vi "PMLambda-Conct Rev B.vi"(0 "FW inTest":u16(ring) items=["WSD Board", "NML Board"], 2 "work buffer":string, 5 "error in":errorcluster, 6 "Supply Cnt":i32=1 min=1 max=5 step=1, 7 "N Systems":i32=1 min=1 max=8 step=1, 8 "COM Ref In":refnum<vi>, 10 "Msg Ref In":refnum<vi>, 11 "Loop Index":i32) -> (14 "Re-conf Lambda?":bool, 15 "Lambda, nm":i32, 19 "error out":errorcluster)   [LabVIEW 2017]
panel:
  # "Inputs"
  # "Outputs"
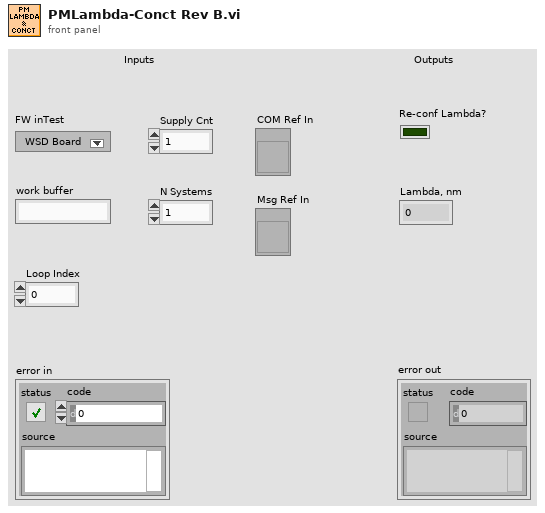
[diagram p1: front panel]
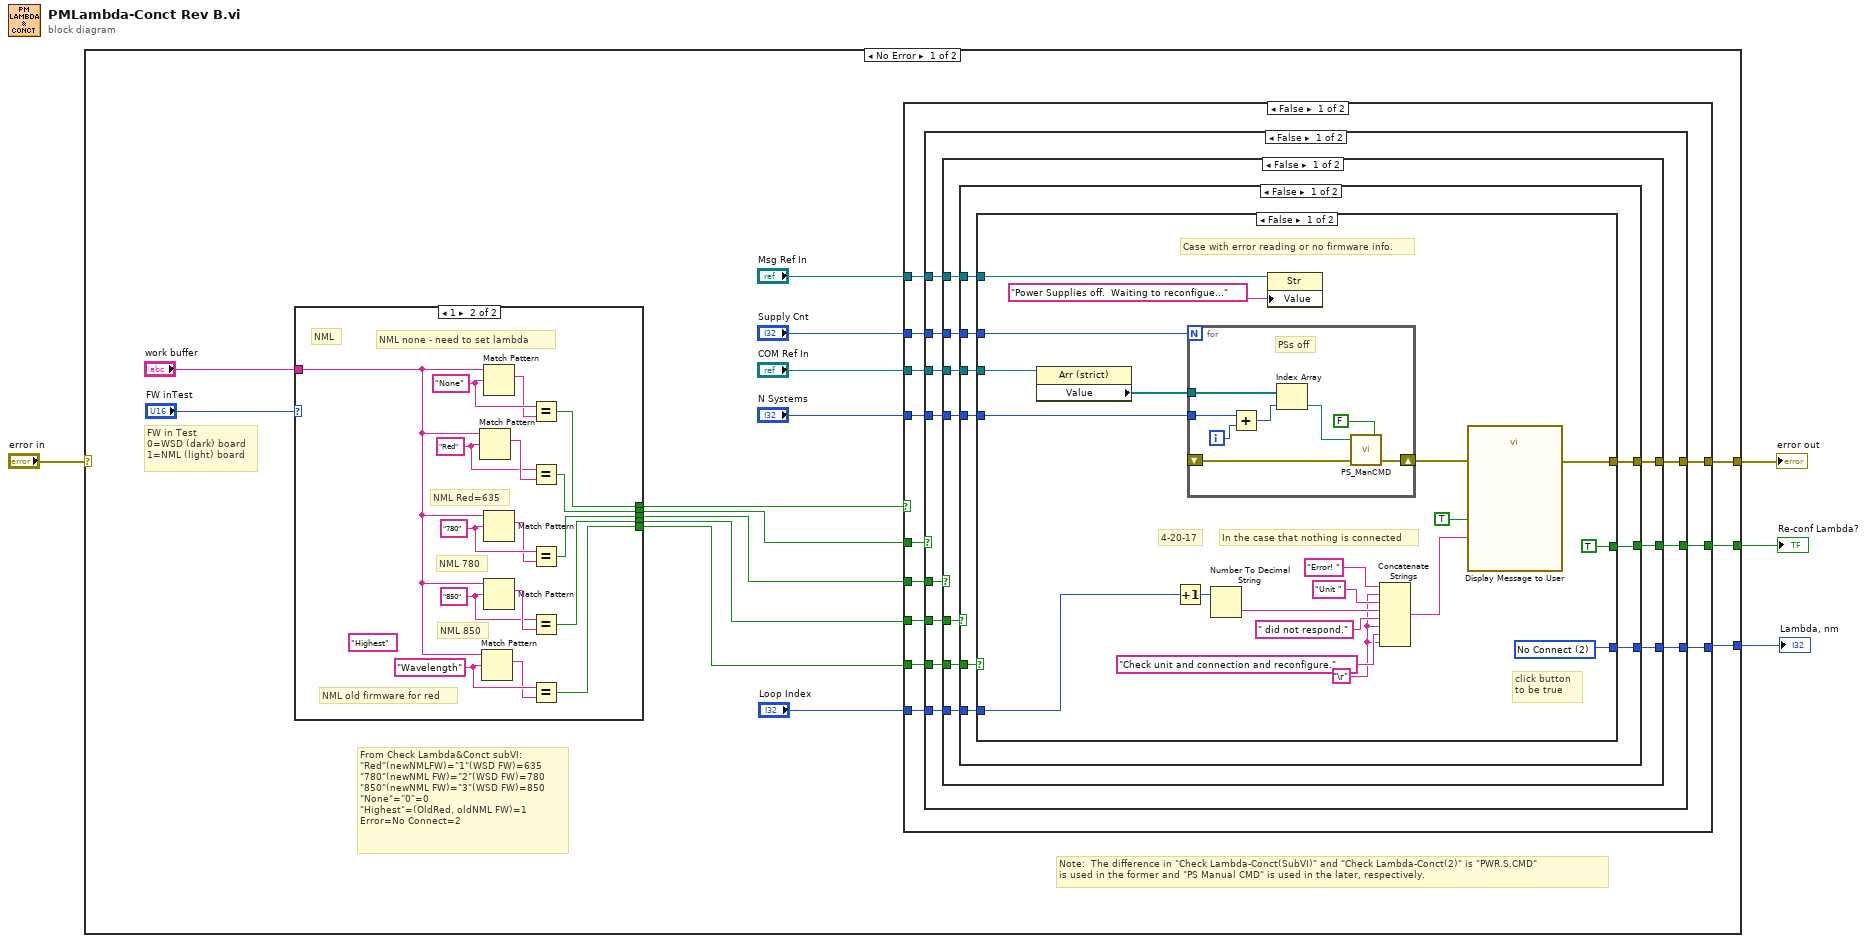
[diagram p0: block diagram]
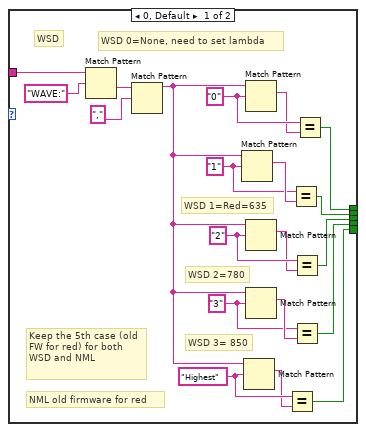
[diagram p2: hidden frame]
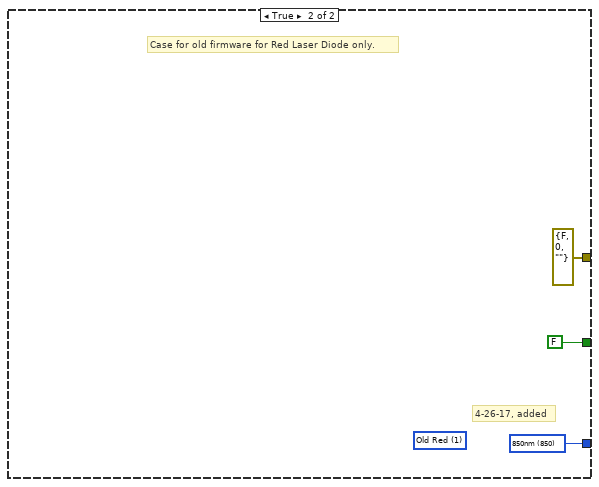
[diagram p3: hidden frame]
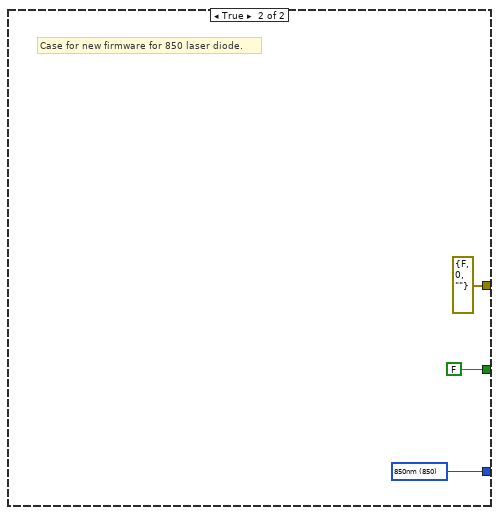
[diagram p4: hidden frame]
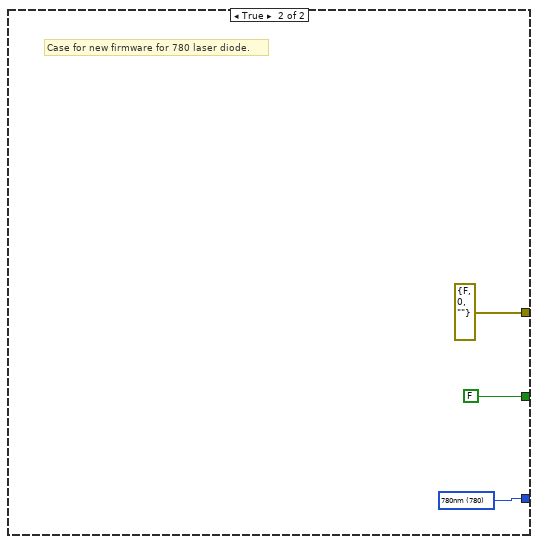
[diagram p5: hidden frame]
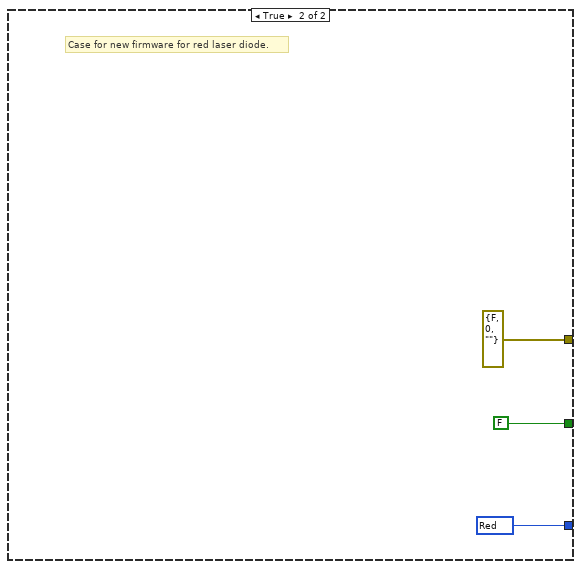
[diagram p6: hidden frame]
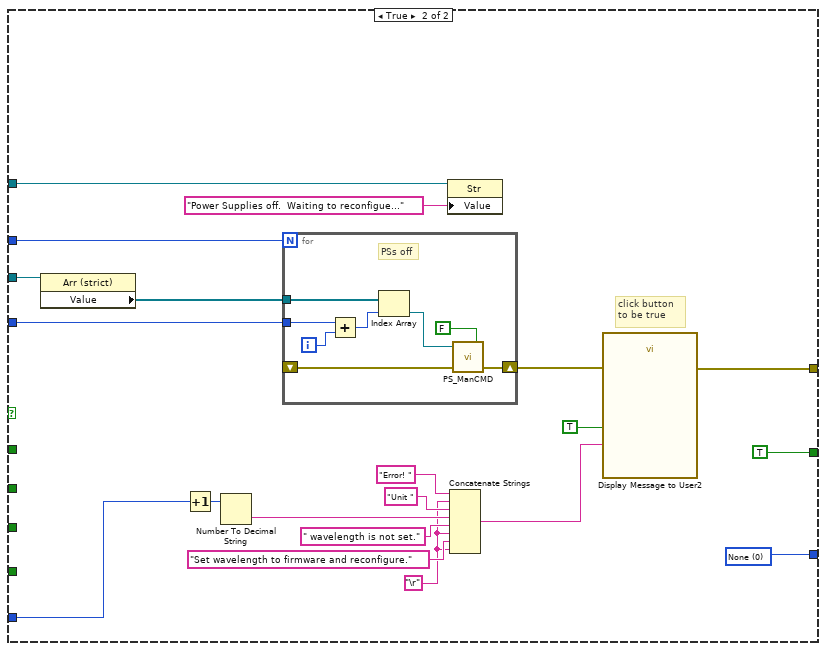
[diagram p7: hidden frame]
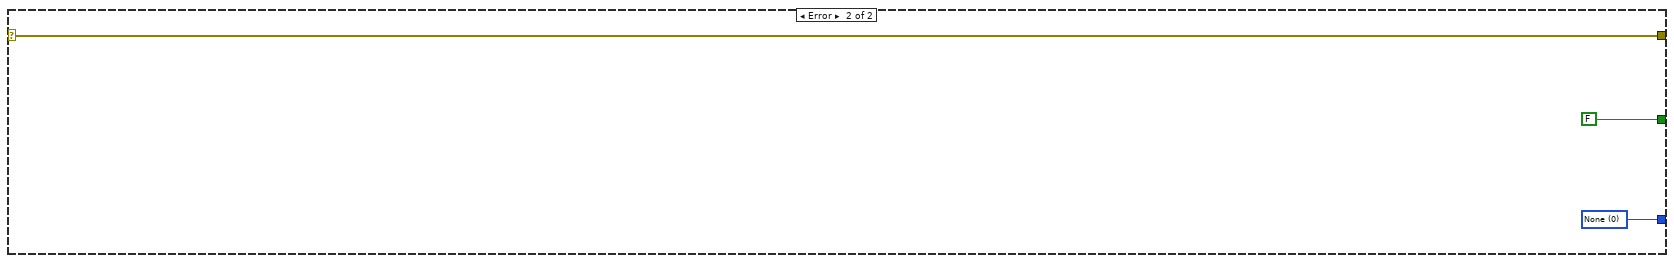
[diagram p8: hidden frame]
diagram:
  n1 = case shown="No Error" "error in" {
    selector: "error in" -> [_ w168]
    tunnel: [w19 FALSE ("Restart Test")] -> w4
    tunnel: [w17 w166] -> w3
    tunnel: [w14 w168] -> w2
    frame No Error {
      # "From Check Lambda&Conct subVI:\n\"Red\"(newNMLFW)=\"1\"(WSD FW)=635\n\"780\"(newNML FW)=\"2\"(WSD FW)=780\n\"850\"(newNML FW)=\"3\"(WSD FW)=850\n\"None\"=\"0\"=0\n\"Highest\"=(OldRed, oldNML FW)=1\nError=No Connect=2"
      # "FW in Test\n0=WSD (dark) board\n1=NML (light) board"
      # "Note:  The difference in \"Check Lambda-Conct(SubVI)\" and \"Check Lambda-Conct(2)\" is \"PWR.S.CMD\" \nis used in the former and \"PS Manual CMD\" is used in the later, respectively."
      n2 = case shown="1" "FW inTest" {
        tunnel: [w25 w45] -> w9
        tunnel: [w24 w44] -> w8
        tunnel: [w23 w43] -> w7
        tunnel: [w22 w42] -> w6
        tunnel: [w21 w41] -> w5
        tunnel: "work buffer" -> [w20 w40]
        frame 0, Default {
          w30 = "Highest" ("regular expression")
          w37 = "3" ("regular expression")
          w36 = "2" ("regular expression")
          w33 = "1" ("regular expression")
          w32 = "0" ("regular expression")
          # "NML old firmware for red"
          # "Keep the 5th case (old FW for red) for both WSD and NML"
          # "WSD"
          # "WSD 3= 850"
          # "WSD 2=780"
          # "WSD 1=Red=635"
          # "WSD 0=None, need to set lambda"
          n3 = Match Pattern(string=w20, regular expression="WAVE:") -> (after substring=w27:string)  [unwired: 1 in, 3 out]
          n4 = Match Pattern(string=w27, regular expression=",") -> (before substring=w39:string)  [unwired: 1 in, 3 out]
          n5 = Match Pattern(string=w39, regular expression=w33) -> (match substring=w34:string)  [unwired: 1 in, 3 out]
          n6 = Match Pattern(string=w39, regular expression=w30) -> (match substring=w29:string)  [unwired: 1 in, 3 out]
          n7 = Match Pattern(string=w39, regular expression=w32) -> (match substring=w31:string)  [unwired: 1 in, 3 out]
          n8 = Match Pattern(string=w39, regular expression=w36) -> (match substring=w35:string)  [unwired: 1 in, 3 out]
          n9 = Match Pattern(string=w39, regular expression=w37) -> (match substring=w38:string)  [unwired: 1 in, 3 out]
          n10 = Equal?(x=w30, y=w29) -> (x = y?=w21:bool)
          n11 = Equal?(x=w33, y=w34) -> (x = y?=w24:bool)
          n12 = Equal?(x=w36, y=w35) -> (x = y?=w23:bool)
          n13 = Equal?(x=w37, y=w38) -> (x = y?=w22:bool)
          n14 = Equal?(x=w32, y=w31) -> (x = y?=w25:bool)
        }
        frame 1 {
          (unwired) "Highest" ("regular expression")
          w47 = "Wavelength" ("regular expression")
          w54 = "850" ("regular expression")
          w53 = "780" ("regular expression")
          w50 = "Red" ("regular expression")
          w49 = "None" ("regular expression")
          # "NML old firmware for red"
          # "NML 850"
          # "NML 780"
          # "NML Red=635"
          # "NML none - need to set lambda"
          # "NML"
          n15 = Match Pattern(string=w40, regular expression=w50) -> (match substring=w51:string)  [unwired: 1 in, 3 out]
          n16 = Match Pattern(string=w40, regular expression=w47) -> (match substring=w46:string)  [unwired: 1 in, 3 out]
          n17 = Match Pattern(string=w40, regular expression=w49) -> (match substring=w48:string)  [unwired: 1 in, 3 out]
          n18 = Match Pattern(string=w40, regular expression=w53) -> (match substring=w52:string)  [unwired: 1 in, 3 out]
          n19 = Match Pattern(string=w40, regular expression=w54) -> (match substring=w55:string)  [unwired: 1 in, 3 out]
          n20 = Equal?(x=w49, y=w48) -> (x = y?=w45:bool)
          n21 = Equal?(x=w50, y=w51) -> (x = y?=w44:bool)
          n22 = Equal?(x=w53, y=w52) -> (x = y?=w43:bool)
          n23 = Equal?(x=w54, y=w55) -> (x = y?=w42:bool)
          n24 = Equal?(x=w47, y=w46) -> (x = y?=w41:bool)
        }
      }
      n25 = case shown="False" w9 {
        tunnel: [w66 w157] -> w17
        tunnel: w8 -> [w67 _]
        tunnel: w7 -> [w65 _]
        tunnel: w6 -> [w64 _]
        tunnel: w5 -> [w63 _]
        tunnel: "Loop Index" -> [w58 w148]
        tunnel: [w62 TRUE ("Restart Test")] -> w19
        tunnel: "COM Ref In" -> [w61 w142]
        tunnel: "Msg Ref In" -> [w60 w141]
        tunnel: [w59 w140] -> w14
        tunnel: "Supply Cnt" -> [w57 w139]
        tunnel: "N Systems" -> [w56 w138]
        frame False {
          n26 = case shown="False" w67 {
            tunnel: [w77 w136] -> w66
            tunnel: w65 -> [w78 _]
            tunnel: w64 -> [w76 _]
            tunnel: w63 -> [w75 _]
            tunnel: [w74 FALSE] -> w62
            tunnel: w61 -> [w73 _]
            tunnel: w60 -> [w72 _]
            tunnel: [w71 errorcluster {"status"=FALSE, "code"=0, "source"=""} ("error out")] -> w59
            tunnel: w58 -> [w70 _]
            tunnel: w57 -> [w69 _]
            tunnel: w56 -> [w68 _]
            frame False {
              n27 = case shown="False" w78 {
                tunnel: [w87 w133] -> w77
                tunnel: w76 -> [w88 _]
                tunnel: w75 -> [w86 _]
                tunnel: [w85 FALSE] -> w74
                tunnel: w73 -> [w84 _]
                tunnel: w72 -> [w83 _]
                tunnel: [w82 errorcluster {"status"=FALSE, "code"=0, "source"=""} ("error out")] -> w71
                tunnel: w70 -> [w81 _]
                tunnel: w69 -> [w80 _]
                tunnel: w68 -> [w79 _]
                frame False {
                  n28 = case shown="False" w88 {
                    tunnel: [w96 w130] -> w87
                    tunnel: w86 -> [w97 _]
                    tunnel: [w95 FALSE] -> w85
                    tunnel: w84 -> [w94 _]
                    tunnel: w83 -> [w93 _]
                    tunnel: [w92 errorcluster {"status"=FALSE, "code"=0, "source"=""} ("error out")] -> w82
                    tunnel: w81 -> [w91 _]
                    tunnel: w80 -> [w90 _]
                    tunnel: w79 -> [w89 _]
                    frame False {
                      n29 = case shown="False" w97 {
                        tunnel: [w108 w127] -> w96
                        tunnel: [TRUE FALSE] -> w95
                        tunnel: w94 -> [w105 _]
                        tunnel: w93 -> [w104 _]
                        tunnel: [w103 errorcluster {"status"=FALSE, "code"=0, "source"=""} ("error out")] -> w92
                        tunnel: w91 -> [w100 _]
                        tunnel: w90 -> [w99 _]
                        tunnel: w89 -> [w98 _]
                        frame False {
                          w108 = 2 items=["None"=0, "Red"=635, "780nm"=780, "850nm"=850, "Old Red"=1, "No Connect"=2]
                          w106 = "\r"
                          # "Case with error reading or no firmware info."
                          # "click button \nto be true"
                          # "In the case that nothing is connected"
                          # "4-20-17"
                          n30 = property class="Arr (strict)"(reference=w105) -> ("Value"=w101:refnum<visa-resource-name>[])  [unwired: 1 in, 2 out]
                          n31 = Increment(x=w100) -> (x+1=w117:i32)
                          n32 = for {
                            N: w99 -> [_]
                            tunnel: w101 -> [w125]
                            shift-right: [w124] -> w102
                            shift-left: _ -> [w123]
                            tunnel: w98 -> [w118]
                            i -> [w120]
                            # "PSs off"
                            n33 = Add(x=w118, y=w120) -> (x+y=w119:i32)
                            n34 = Index Array(array=w125, index=w119) -> (element=w121:refnum<visa-resource-name>)
                            n35 = call "PS_ManCMD.vi"("Power Sup: T-On/F-Off"=FALSE, "error in"=w123, "VISA resource name"=w121) -> ("error out"=w124:errorcluster)  [unwired: 2 in]
                          }
                          n36 = Number To Decimal String(number=w117) -> (decimal integer string=w113:string)  [unwired: 1 in]
                          n37 = property class="Str"(reference=w104, "Value"="Power Supplies off.  Waiting to reconfigue..." ("Msg")) -> ()  [unwired: 1 in, 2 out]
                          n38 = Concatenate Strings("Error! " ("string"), w106, "Unit " ("string"), w113, " did not respond." ("string"), w106, "Check unit and connection and reconfigure." ("string"), w106) -> (w114:string)
                          n39 = call "Display Message to User"("error in (no error)"=w102, "Enable"=TRUE, "Message"=w114) -> ("error out"=w103:errorcluster)  [unwired: 7 in, 1 out]
                        }
                        frame True {
                          (unwired) 1 items=["None"=0, "Red"=635, "780nm"=780, "850nm"=850, "Old Red"=1, "No Connect"=2]
                          w127 = 850 items=["None"=0, "Red"=635, "780nm"=780, "850nm"=850, "Old Red"=1, "No Connect"=2]
                          # "Case for old firmware for Red Laser Diode only."
                          # "4-26-17, added"
                        }
                      }
                    }
                    frame True {
                      w130 = 850 items=["None"=0, "Red"=635, "780nm"=780, "850nm"=850, "Old Red"=1, "No Connect"=2]
                      # "Case for new firmware for 850 laser diode."
                    }
                  }
                }
                frame True {
                  w133 = 780 items=["None"=0, "Red"=635, "780nm"=780, "850nm"=850, "Old Red"=1, "No Connect"=2]
                  # "Case for new firmware for 780 laser diode."
                }
              }
            }
            frame True {
              w136 = 635 items=["None"=0, "Red"=635, "780nm"=780, "850nm"=850, "Old Red"=1, "No Connect"=2]
              # "Case for new firmware for red laser diode."
            }
          }
        }
        frame True {
          w143 = "\r"
          w157 = 0 items=["None"=0, "Red"=635, "780nm"=780, "850nm"=850, "Old Red"=1, "No Connect"=2]
          # "click button \nto be true"
          n40 = property class="Arr (strict)"(reference=w142) -> ("Value"=w147:refnum<visa-resource-name>[])  [unwired: 1 in, 2 out]
          n41 = Increment(x=w148) -> (x+1=w156:i32)
          n42 = Number To Decimal String(number=w156) -> (decimal integer string=w152:string)  [unwired: 1 in]
          n43 = for {
            N: w139 -> [_]
            tunnel: w147 -> [w165]
            shift-right: [w164] -> w146
            shift-left: _ -> [w163]
            tunnel: w138 -> [w158]
            i -> [w160]
            # "PSs off"
            n44 = Add(x=w158, y=w160) -> (x+y=w159:i32)
            n45 = Index Array(array=w165, index=w159) -> (element=w161:refnum<visa-resource-name>)
            n46 = call "PS_ManCMD.vi"("Power Sup: T-On/F-Off"=FALSE, "error in"=w163, "VISA resource name"=w161) -> ("error out"=w164:errorcluster)  [unwired: 2 in]
          }
          n47 = property class="Str"(reference=w141, "Value"="Power Supplies off.  Waiting to reconfigue..." ("Msg")) -> ()  [unwired: 1 in, 2 out]
          n48 = Concatenate Strings("Error! " ("string"), w143, "Unit " ("string"), w152, " wavelength is not set." ("string"), w143, "Set wavelength to firmware and reconfigure." ("string"), w143) -> (w153:string)
          n49 = call "Display Message to User2"("error in (no error)"=w146, "Enable"=TRUE, "Message"=w153) -> ("error out"=w140:errorcluster)  [unwired: 7 in, 1 out]
        }
      }
    }
    frame Error {
      w166 = 0 items=["None"=0, "Red"=635, "780nm"=780, "850nm"=850, "Old Red"=1, "No Connect"=2]
    }
  }
  "Re-conf Lambda?" <- w4
  "Lambda, nm" <- w3
  "error out" <- w2
